vi "Cal Inst - Initialize.vi"(8 "error in (no error)":errorcluster, 9 "Voltage Level (0V)":dbl, 10 "Serial Configuration":cluster{"Baud Rate":u32, "Flow Control":u16}={"Baud Rate"=460800, "Flow Control"=0} {"Flow Control" items=["None", "XON/XOFF", "RTS/CTS", "XON/XOFF & RTS/CTS", "DTR/DSR", "XON/XOFF & DTR/DSR"]; "Baud Rate" items=["9600"=9600, "19200"=19200, "38400"=38400, "57600"=57600, "115200"=115200, "230400"=230400, "460800"=460800]}, 11 "VISA Refnum in":refnum<visa-resource-name>) -> (0 "error out":errorcluster, 3 "VISA Refnum out":refnum<visa-resource-name>)   [LabVIEW 2013, in "Cal Inst Acquisition.lvlib"]
uses:
  Cal Inst Acquisition.lvlib
  Libraries/California Instruments iX Series/California Instruments iX Series.lvlib
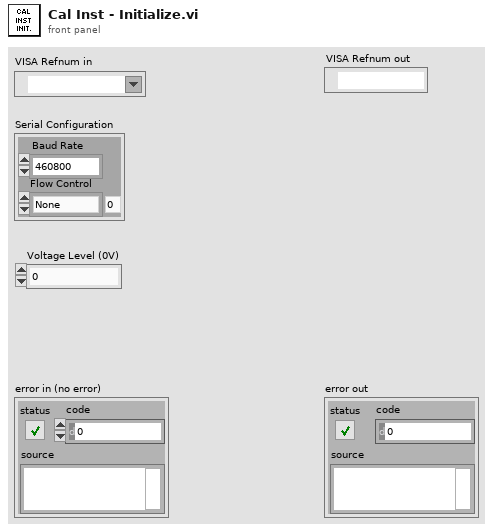
[diagram p1: front panel]
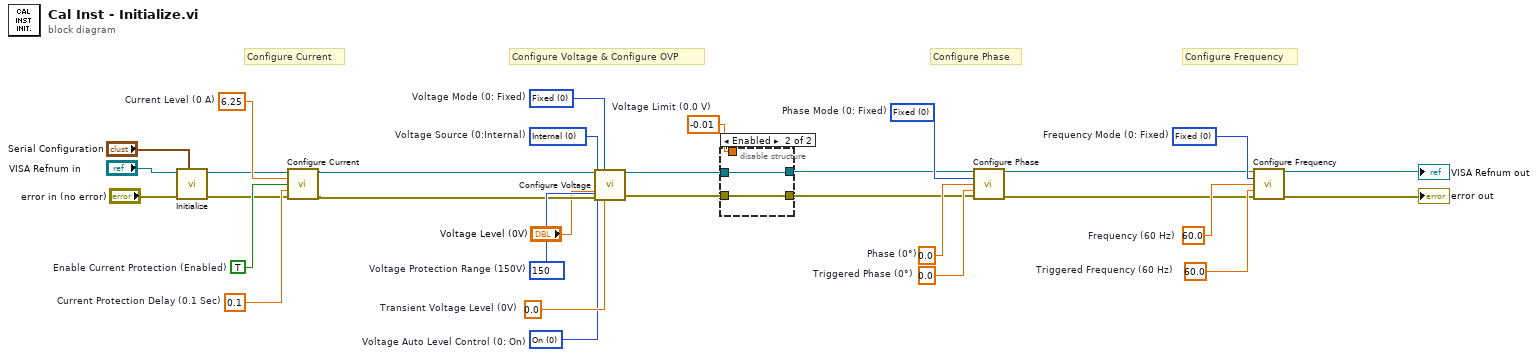
[diagram p0: block diagram]
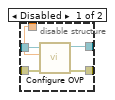
[diagram p2: hidden frame]
diagram:
  w14 = 60.0  # Triggered Frequency (60 Hz)
  w13 = 60.0  # Frequency (60 Hz)
  w12 = 0 items=["Fixed", "Step", "Pulse", "List", "Sense", "External"]  # Frequency Mode (0: Fixed)
  w17 = 0.0  # Triggered Phase (0°)
  w16 = 0.0  # Phase (0°)
  w15 = 0 items=["Fixed", "Step", "Pulse", "List"]  # Phase Mode (0: Fixed)
  w25 = -0.01  # Voltage Limit (0.0 V)
  w22 = u16 150 items=["150"=150, "300"=300]  # Voltage Protection Range (150V)
  w19 = u16 0 items=["On", "Off", "Regulation"]  # Voltage Auto Level Control (0: On)
  w20 = u16 0 items=["Internal", "External"]  # Voltage Source (0:Internal)
  w18 = 0 items=["Fixed", "Step", "Pulse", "List"]  # Voltage Mode (0: Fixed)
  w21 = 0.0  # Transient Voltage Level (0V)
  w28 = 0.1  # Current Protection Delay (0.1 Sec)
  w27 = TRUE  # Enable Current Protection (Enabled)
  w26 = 6.25  # Current Level (0 A)
  # "Configure Frequency"
  # "Configure Phase"
  # "Configure Voltage & Configure OVP"
  # "Configure Current"
  n1 = call "Initialize.vi"("Serial Configuration"="Serial Configuration", "error in (no error)"="error in (no error)", "VISA resource name"="VISA Refnum in") -> ("error out"=w4:errorcluster, "VISA resource name out"=w5:refnum<visa-resource-name>)  [unwired: 7 in]
  n2 = call "Configure Current.vi"("VISA resource name"=w5, "Current Level (0 A)"=w26, "Enable Current Protection (Enabled)"=w27, "Current Protection Delay (0.1 Sec)"=w28, "error in (no error)"=w4) -> ("VISA resource name out"=w11:refnum<visa-resource-name>, "error out"=w10:errorcluster)  [unwired: 9 in]
  n3 = call "Configure Voltage.vi"("VISA resource name"=w11, "Voltage Mode (0: Fixed)"=w18, "Voltage Auto Level Control (0: On)"=w19, "Voltage Source (0:Internal)"=w20, "Voltage Level (0V)"="Voltage Level (0V)", "error in (no error)"=w10, "Transient Voltage Level (0V)"=w21, "Voltage Protection Range (150V)"=w22) -> ("VISA resource name out"=w23:refnum<visa-resource-name>, "error out"=w24:errorcluster)  [unwired: 6 in]
  n4 = disable-structure shown="Enabled" {
    disable-tunnel: w23 -> [w36 w38]
    disable-tunnel: w24 -> [w35 w37]
    disable-tunnel: w25 -> [w34 _]
    disable-tunnel: [w33 w38] -> w9
    disable-tunnel: [w32 w37] -> w8
    frame Disabled {
      n5 = call "Configure OVP.vi"("error in (no error)"=w35, "Voltage Limit (0.0 V)"=w34, "VISA resource name"=w36) -> ("error out"=w32:errorcluster, "VISA resource name out"=w33:refnum<visa-resource-name>)  [unwired: 7 in]
    }
    frame Enabled {
    }
  }
  n6 = call "Configure Phase.vi"("VISA resource name"=w9, "Phase Mode (0: Fixed)"=w15, "Phase (0°)"=w16, "Triggered Phase (0°)"=w17, "error in (no error)"=w8) -> ("VISA resource name out"=w7:refnum<visa-resource-name>, "error out"=w6:errorcluster)  [unwired: 9 in]
  n7 = call "Configure Frequency.vi"("VISA resource name"=w7, "Frequency Mode (0: Fixed)"=w12, "Frequency (60 Hz)"=w13, "Triggered Frequency (60 Hz)"=w14, "error in (no error)"=w6) -> ("VISA resource name out"=→"VISA Refnum out":refnum<visa-resource-name>, "error out"=→"error out":errorcluster)  [unwired: 9 in]
